vi "GetPaths.vi"(8 "error in (no error)":errorcluster, 11 "path":path) -> (0 "error out":errorcluster, 3 "All Files in Dir":path[](array[path]))   [LabVIEW 2023]
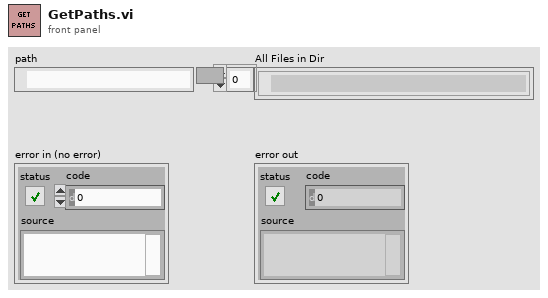
[diagram p1: front panel]
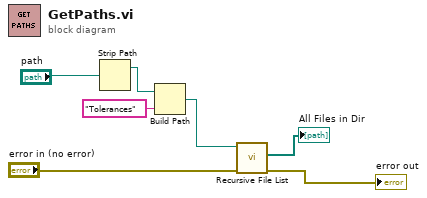
[diagram p0: block diagram]
diagram:
  n1 = Strip Path(path="path") -> (stripped path=w3:path)  [unwired: 1 out]
  n2 = Build Path(base path=w3, name or relative path="Tolerances") -> (appended path=w4:path)
  n3 = call <vilib>:"Recursive File List.vi"("error in (no error)"="error in (no error)", "Folder Path"=w4) -> ("error out"=→"error out":errorcluster, "All Files in Dir"=→"All Files in Dir":path[])  [unwired: 5 in, 3 out]
